vi "LVtest.vi"() -> ()   [LabVIEW 2018]
uses:
  <vilib>/Instr/_visa.llb/VISA Configure Serial Port (Instr).vi
  milGrabber/vs2017/x64/Debug/milGrabberInterface.dll
panel:
  out "size(s)":i32[](array[numeric])
  out "Higher image":u16[][](graph)
  out "Lower image":u16[][](graph)
  in  "index (row) 2":i32
  out "frame size":i64
  in  "index (row)":i32
  out "get":i32
  out "error out 4":errorcluster
  out "read buffer":string
  out "error out 3":errorcluster
  out "error out 2":errorcluster
  out "error out":errorcluster
  out "Intensity Graph":u8[][](graph)
  out "destroy":i32
  out "Start":i32
  out "int":i32
  # "775 * 385 * 4 = 1193500"
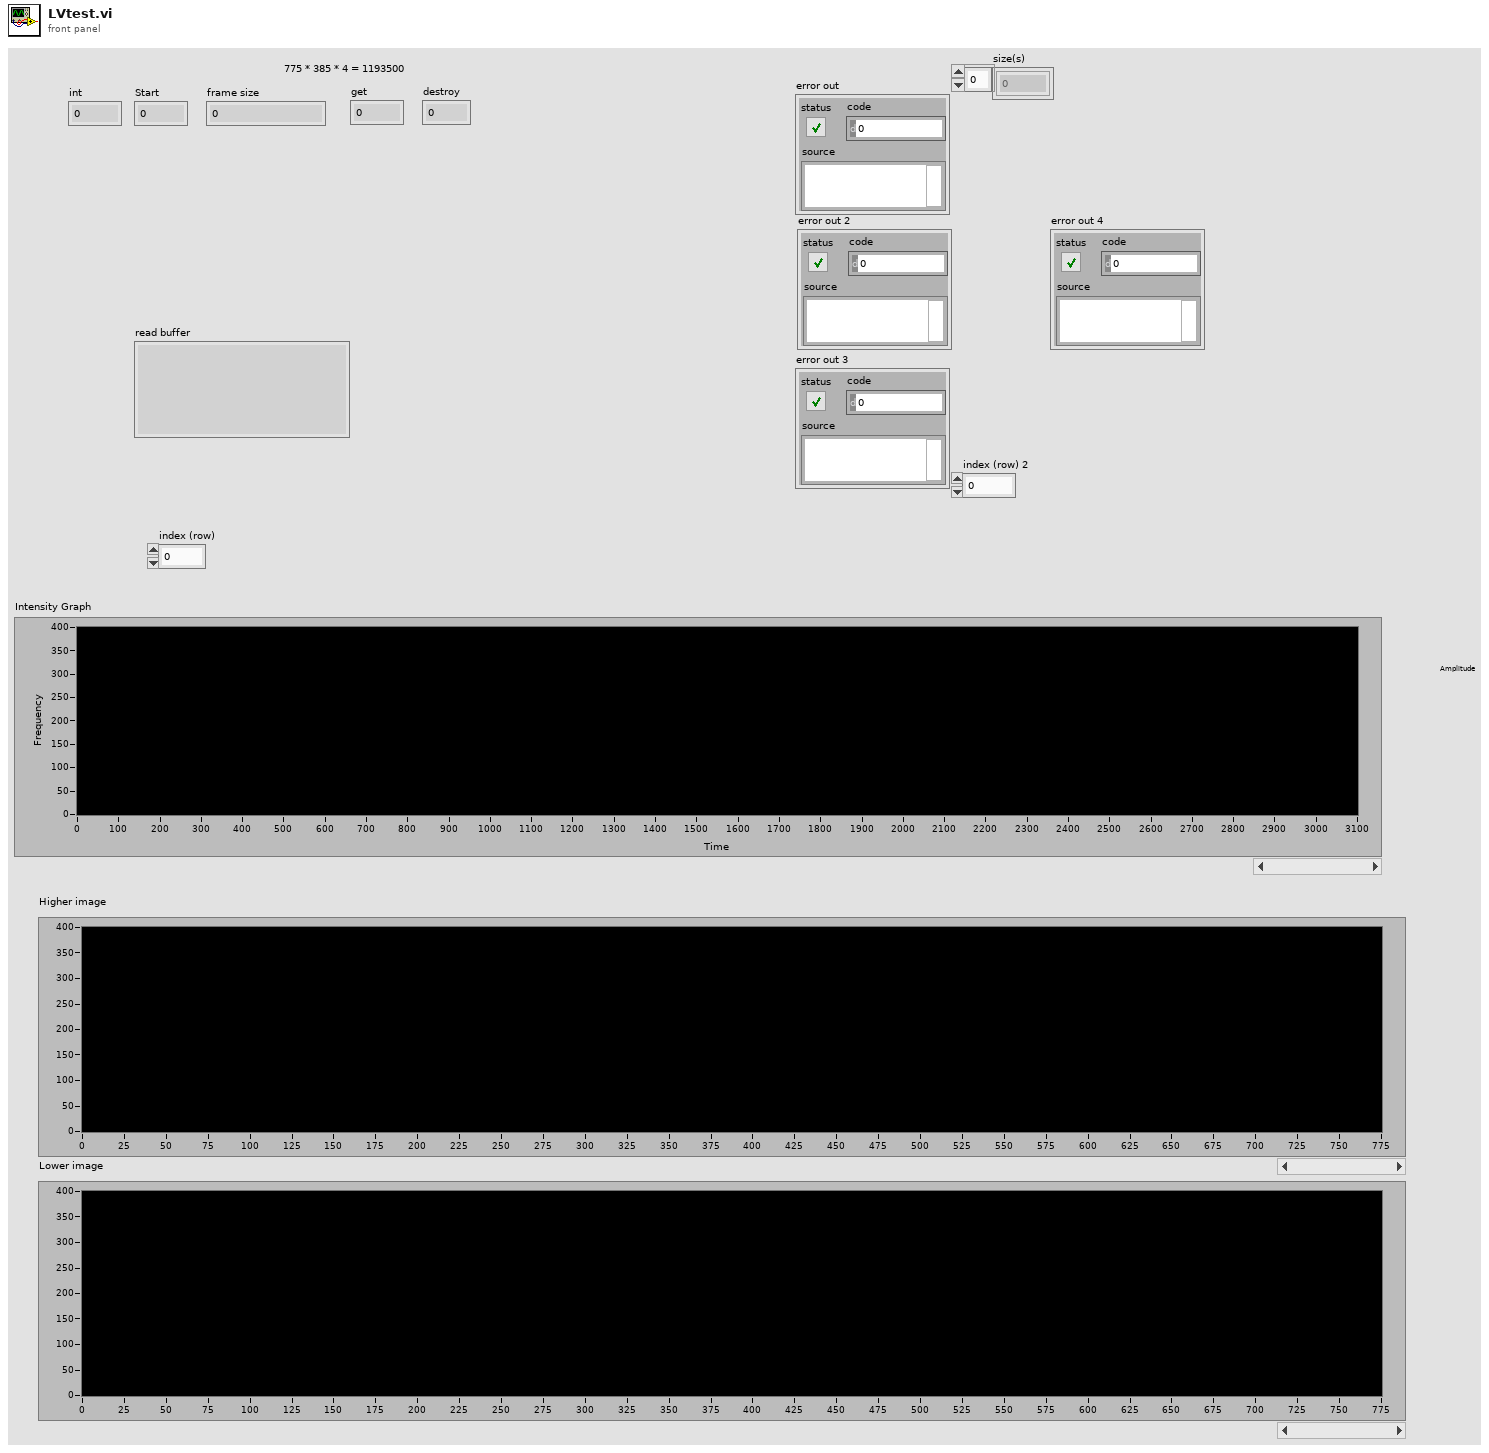
[diagram p1: front panel]
types:
  T1 = enum16{"big-endian, network order", "native, host order", "little-endian"}
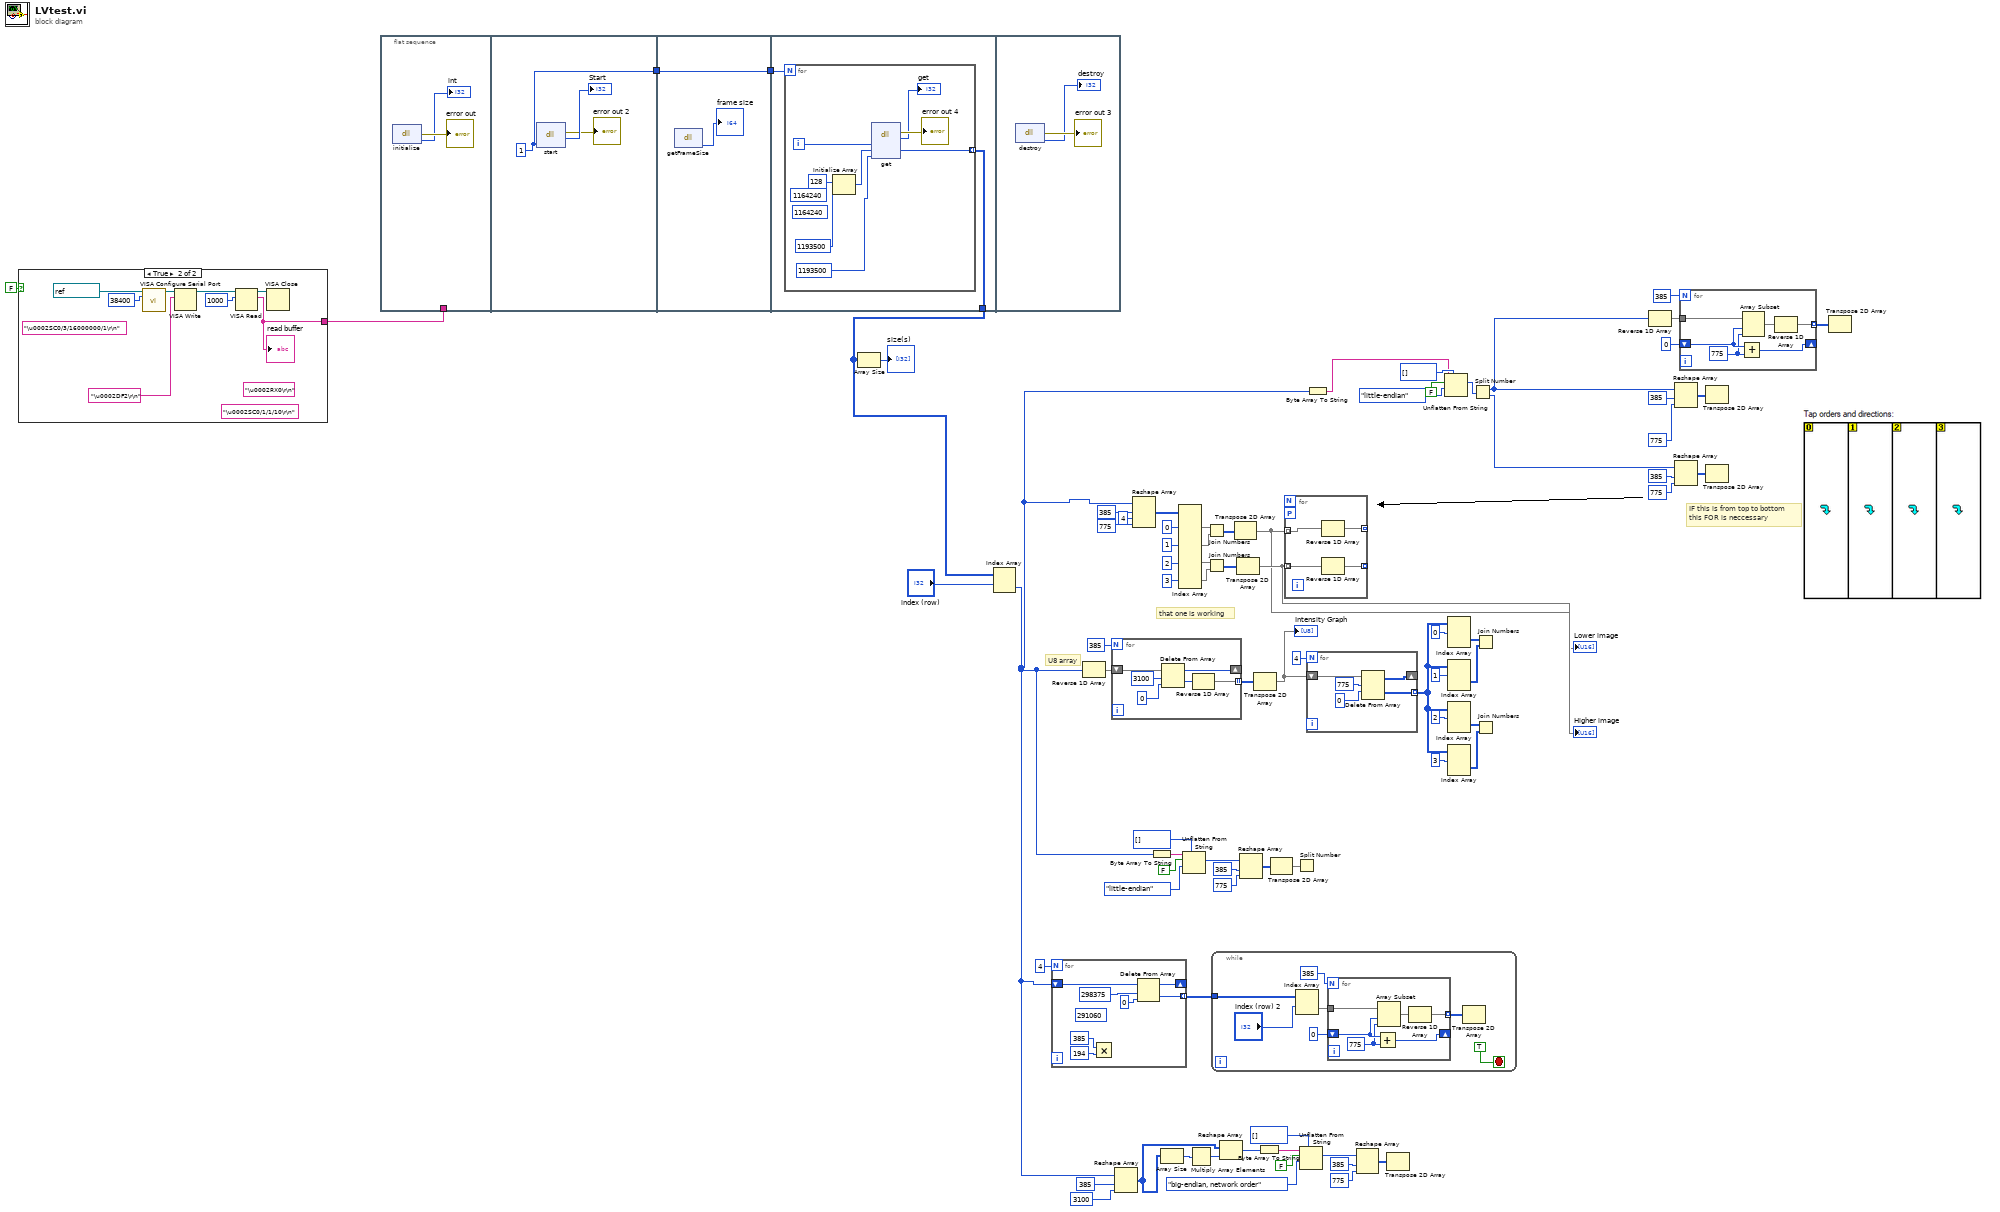
[diagram p0: block diagram]
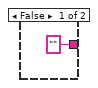
[diagram p2: hidden frame]
diagram:
  # "U8 array"
  # "that one is working"
  # "IF this is from top to bottom \nthis FOR is neccessary"
  n1 = case shown="True" FALSE {
    tunnel: ["" ("read buffer") w83] -> w79
    frame False {
    }
    frame True {
      (unwired) "\u0002SC0/1/1/10\r\n" ("format string")
      (unwired) "\u0002RX0\r\n" ("format string")
      (unwired) "\u0002SC0/3/16000000/1\r\n" ("format string")
      n2 = call-poly "VISA Configure Serial Port"("VISA resource name"=refnum<visa-resource-name> "COM3", "baud rate (9600)"=u32 38400) -> ("VISA resource name out"=w87:refnum<visa-resource-name>)  [unwired: 12 in, 1 out]
      n3 = VISA Write(VISA resource name=w87, write buffer="\u0002DF2\r\n" ("format string")) -> (VISA resource name out=w86:refnum<visa-resource-name>)  [unwired: 1 in, 2 out]
      n4 = VISA Read(VISA resource name=w86, byte count=u32 1000) -> (VISA resource name out=w85:refnum<visa-resource-name>, read buffer=w83:string)  [unwired: 1 in, 2 out]
      "read buffer" <- w83
      n5 = VISA Close(VISA resource name=w85) -> ()  [unwired: 1 in, 1 out]
    }
  }
  n6 = flat-sequence {
    tunnel: [w90] -> _
    tunnel: w79 -> [w90]
    tunnel: [w93] -> w78
    tunnel: w78 -> [w97]
    tunnel: [w97] -> w77
    tunnel: w77 -> [w99]
    tunnel: [w98] -> w33
    frame #0 {
      n7 = dll-call lib="C:/Users/Kinga/Desktop/Matrox/Testy/milGrabber/vs2017/x64/Debug/milGrabberInterface.dll" fn="initialize"() -> (error out=→"error out":errorcluster, "int"=→"int":i32)  [unwired: 3 in, 1 out]
    }
    frame #1 {
      w93 = i16 1 ("grabFramesNo")
      n8 = dll-call lib="C:/Users/Kinga/Desktop/Matrox/Testy/milGrabber/vs2017/x64/Debug/milGrabberInterface.dll" fn="start"("grabFramesNo"=w93) -> (error out=→"error out 2":errorcluster, "int"=→"Start":i32)  [unwired: 4 in, 1 out]
    }
    frame #2 {
      n9 = dll-call lib="C:/Users/Kinga/Desktop/Matrox/Testy/milGrabber/vs2017/x64/Debug/milGrabberInterface.dll" fn="getFrameSize"() -> ("int"=→"frame size":i64)  [unwired: 3 in, 2 out]
    }
    frame #3 {
      n10 = for {
        N: w99 -> [_]
        tunnel: [w102] -> w98 mode=indexing
        i -> [w103]
        (unwired) 1164240 ("out_size")
        (unwired) 1164240 ("dimension size")
        n11 = Initialize Array(u8 128 ("element"), 1193500 ("out_size")) -> (w104:u8[])
        n12 = dll-call lib="C:/Users/Kinga/Desktop/Matrox/Testy/milGrabber/vs2017/x64/Debug/milGrabberInterface.dll" fn="get"("frameNum"=w103, "out_buf"=w104, "out_size"=1193500 ("dimension size")) -> (error out=→"error out 4":errorcluster, "int"=→"get":i32, "out_buf"=w102:u8[])  [unwired: 5 in, 1 out]
      }
    }
    frame #4 {
      n13 = dll-call lib="C:/Users/Kinga/Desktop/Matrox/Testy/milGrabber/vs2017/x64/Debug/milGrabberInterface.dll" fn="destroy"() -> (error out=→"error out 3":errorcluster, "int"=→"destroy":i32)  [unwired: 3 in, 1 out]
    }
  }
  n14 = Array Size(array=w33) -> (size(s)=→"size(s)":i32[])
  n15 = Index Array(array=w33, index (row)="index (row)") -> (element=w39:u8[])  [unwired: 1 in]
  n16 = for {
    N: 4 -> [_]
    shift-right: [w116] -> _
    shift-left: w39 -> [w111]
    tunnel: [w112] -> w50 mode=indexing
    (unwired) 291060 ("length")
    n17 = Multiply(x=385, y=194 ("length")) -> ()  [unwired: 1 out]
    n18 = Delete From Array(array=w111, length=298375, index=0) -> (deleted portion=w112:u8[], array with subset deleted=w116:u8[])
  }
  n19 = Reverse 1D Array(array=w39) -> (reversed array=w28:u8[])
  n20 = for {
    N: 385 -> [_]
    tunnel: [w122] -> w29 mode=indexing
    shift-right: [w119] -> _
    shift-left: w28 -> [w120]
    n21 = Delete From Array(array=w120, length=3100, index=0) -> (deleted portion=w121:u8[], array with subset deleted=w119:u8[])
    n22 = Reverse 1D Array(array=w121) -> (reversed array=w122:u8[])
  }
  n23 = Reshape Array(w39, 385 ("dimension size"), 3100 ("dimension size")) -> (w51:u8[][])
  n24 = Reshape Array(w39, 385, 4 ("dimension size"), 775 ("length")) -> (w4:u8[][][])
  n25 = Byte Array To String(unsigned byte array=w39) -> (string=w57:string)
  n26 = Array Size(array=w51) -> (size(s)=w73:i32[])
  n27 = Index Array(array=w4, index (dim 1) #1=0 ("disabled index (row)"), index (dim 1) #2=1 ("index (row)"), index (dim 1) #3=2 ("disabled index (row)"), index (dim 1) #4=3 ("index (row)")) -> (element #1=w15:u8[][], element #2=w10:u8[][], element #3=w9:u8[][], element #4=w8:u8[][])  [unwired: 8 in]
  n28 = Unflatten From String(type=u32[] [] ("U32 Array"), binary string=w57, data includes array or string size? (T)=FALSE, byte order (0:big-endian, network order)=T1."little-endian") -> (value=w52:u32[])  [unwired: 1 in, 2 out]
  n29 = Multiply Array Elements(1:w73) -> (0:w74:i32)
  n30 = Join Numbers(hi=w15, lo=w10) -> ((hi.lo)=w3:u16[][])
  n31 = Join Numbers(hi=w9, lo=w8) -> ((hi.lo)=w7:u16[][])
  n32 = while {
    tunnel: w50 -> [w129]
    stop <- TRUE stop-if-true
    n33 = Index Array(array=w129, index (row)="index (row) 2") -> (element=w125:u8[])  [unwired: 1 in]
    n34 = for {
      N: 385 -> [_]
      tunnel: w125 -> [w134]
      tunnel: [w135] -> w124 mode=indexing
      shift-right: [w131] -> _
      shift-left: 0 -> [w132]
      w130 = 775 ("length")
      n35 = Add(x=w132, y=w130) -> (x+y=w131:i32)
      n36 = Array Subset(array=w134, index=w132, length=w130) -> (w133:u8[])
      n37 = Reverse 1D Array(array=w133) -> (reversed array=w135:u8[])
    }
    n38 = Transpose 2D Array(2D array=w124) -> ()  [unwired: 1 out]
  }
  n39 = Reshape Array(w51, w74) -> (w72:u8[])
  n40 = Transpose 2D Array(2D array=w3) -> (transposed array=w1:u16[][])
  "Lower image" <- w1
  n41 = Transpose 2D Array(2D array=w7) -> (transposed array=w2:u16[][])
  "Higher image" <- w2
  n42 = Reshape Array(w52, 385 ("dimension size"), 775 ("dimension size")) -> (w54:u32[][])
  n43 = Transpose 2D Array(2D array=w29) -> (transposed array=w26:u8[][])
  "Intensity Graph" <- w26
  n44 = Byte Array To String(unsigned byte array=w72) -> (string=w71:string)
  n45 = Transpose 2D Array(2D array=w54) -> (transposed array=w48:u32[][])
  n46 = for {
    tunnel: w1 -> [w139] mode=indexing
    tunnel: [w138] -> _ mode=indexing
    tunnel: w2 -> [w137] mode=indexing
    tunnel: [w136] -> _ mode=indexing
    workers-P: _ -> [_]
    n47 = Reverse 1D Array(array=w139) -> (reversed array=w138:u16[])
    n48 = Reverse 1D Array(array=w137) -> (reversed array=w136:u16[])
  }
  n49 = Split Number(x=w48) -> ()  [unwired: 2 out]
  n50 = Unflatten From String(type=u32[] [] ("U32 Array"), binary string=w71, data includes array or string size? (T)=FALSE, byte order (0:big-endian, network order)=T1."big-endian, network order") -> (value=w64:u32[])  [unwired: 1 in, 2 out]
  n51 = Byte Array To String(unsigned byte array=w39) -> (string=w35:string)
  n52 = for {
    N: 4 -> [_]
    shift-right: [w144] -> _
    shift-left: w26 -> [w142]
    tunnel: [w143] -> w19 mode=indexing
    n53 = Delete From Array(array=w142, length=775, index (row)=0) -> (deleted portion=w143:u8[][], array with subset deleted=w144:u8[][])  [unwired: 1 in]
  }
  n54 = Reshape Array(w64, 385 ("dimension size"), 775 ("dimension size")) -> (w65:u32[][])
  n55 = Transpose 2D Array(2D array=w65) -> ()  [unwired: 1 out]
  n56 = Unflatten From String(type=u32[] [] ("U32 Array"), binary string=w35, data includes array or string size? (T)=FALSE, byte order (0:big-endian, network order)=T1."little-endian") -> (value=w34:u32[])  [unwired: 1 in, 2 out]
  n57 = Index Array(array=w19, index (dim 0)=0 ("index (page)")) -> (element=w23:u8[][])  [unwired: 2 in]
  n58 = Index Array(array=w19, index (dim 0)=1 ("index (page)")) -> (element=w22:u8[][])  [unwired: 2 in]
  n59 = Index Array(array=w19, index (dim 0)=2 ("index (page)")) -> (element=w20:u8[][])  [unwired: 2 in]
  n60 = Index Array(array=w19, index (dim 0)=3 ("index (page)")) -> (element=w21:u8[][])  [unwired: 2 in]
  n61 = Split Number(x=w34) -> (hi(x)=w41:u16[], lo(x)=w49:u16[])
  n62 = Join Numbers(hi=w23, lo=w22) -> ()  [unwired: 1 out]
  n63 = Join Numbers(hi=w20, lo=w21) -> ()  [unwired: 1 out]
  n64 = Reverse 1D Array(array=w41) -> (reversed array=w40:u16[])
  n65 = Reshape Array(w41, 385 ("dimension size"), 775 ("dimension size")) -> (w47:u16[][])
  n66 = Reshape Array(w49, 385 ("dimension size"), 775 ("dimension size")) -> (w53:u16[][])
  n67 = for {
    N: 385 -> [_]
    tunnel: w40 -> [w149]
    tunnel: [w150] -> w42 mode=indexing
    shift-right: [w146] -> _
    shift-left: 0 -> [w147]
    w145 = 775 ("length")
    n68 = Add(x=w147, y=w145) -> (x+y=w146:i32)
    n69 = Array Subset(array=w149, index=w147, length=w145) -> (w148:u16[])
    n70 = Reverse 1D Array(array=w148) -> (reversed array=w150:u16[])
  }
  n71 = Transpose 2D Array(2D array=w47) -> ()  [unwired: 1 out]
  n72 = Transpose 2D Array(2D array=w53) -> ()  [unwired: 1 out]
  n73 = Transpose 2D Array(2D array=w42) -> ()  [unwired: 1 out]
